vi "Has time elapsed.vi"(8 "error in (no error)":errorcluster, 10 "Time target":dbl format="%#_13g", 11 "Action":enum16{"Reset", "Get", "Get difference"}(ring)=enum."Get difference") -> (0 "error out":errorcluster, 2 "Time elapsed":dbl format="%#_13g", 3 "Time elapsed?":bool)   [LabVIEW 2025]
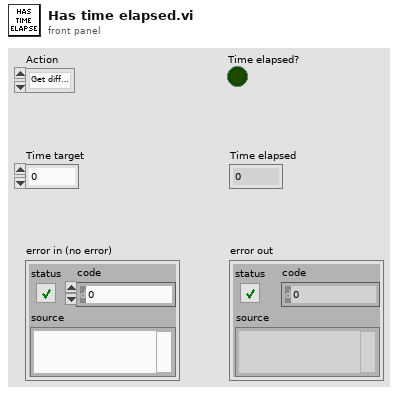
[diagram p1: front panel]
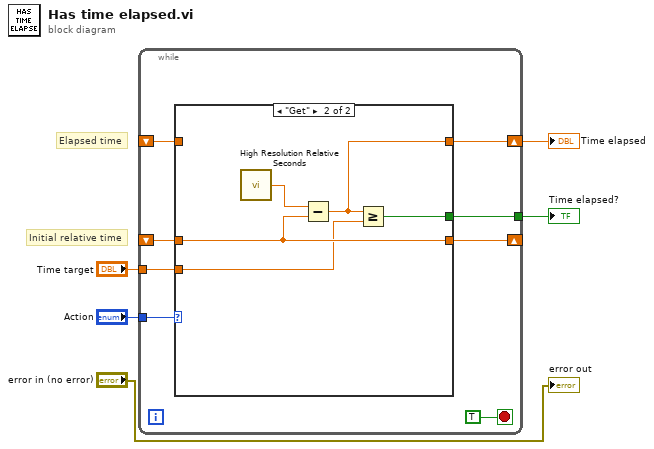
[diagram p0: block diagram]
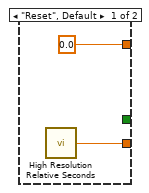
[diagram p2: hidden frame]
diagram:
  # "Initial relative time"
  # "Elapsed time"
  n1 = while {
    tunnel: "Action" -> [w12]
    shift-right: [w10] -> w4
    shift-left: _ -> [w11]
    tunnel: "Time target" -> [w9]
    shift-right: [w8] -> _
    shift-left: _ -> [w7]
    tunnel: [w6] -> w2
    stop <- TRUE stop-if-true
    n2 = case shown="\"Get\"" w12 {
      tunnel: w11 -> [_ _]
      tunnel: [0.0 w16] -> w10
      tunnel: w9 -> [_ w18]
      tunnel: [w14 w19] -> w8
      tunnel: w7 -> [_ w19]
      tunnel: [_ w17] -> w6
      frame "Reset", Default {
        n3 = call <vilib>:"High Resolution Relative Seconds.vi"() -> ("relative seconds"=w14:dbl)
      }
      frame "Get" {
        n4 = call <vilib>:"High Resolution Relative Seconds.vi"() -> ("relative seconds"=w20:dbl)
        n5 = Subtract(x=w20, y=w19) -> (x-y=w16:dbl)
        n6 = Greater Or Equal?(x=w16, y=w18) -> (x >= y?=w17:bool)
      }
    }
  }
  "Time elapsed" <- w4
  "Time elapsed?" <- w2
  "error out" <- "error in (no error)"
